vi "RemoveClassesFromTypeDescriptor.vi"(1 "type descriptor":u8[](array[numeric]) format="%x", 3 "replace type desc":u8[](array[numeric])) -> (15 "type descriptor out":u8[](array[numeric]), 18 "type descriptor parsed out":cluster{"TypeDescr":u8[], "Class":bool}[](array[cluster]))   [LabVIEW 2017, in "G#DebugServer.lvclass"]
uses:
  <vilib>/addons/_AddQ/G#DebugServer/G#DebugServer.lvclass
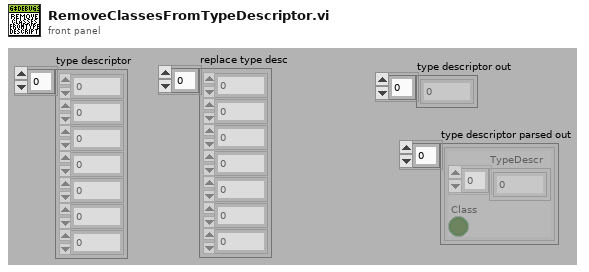
[diagram p1: front panel]
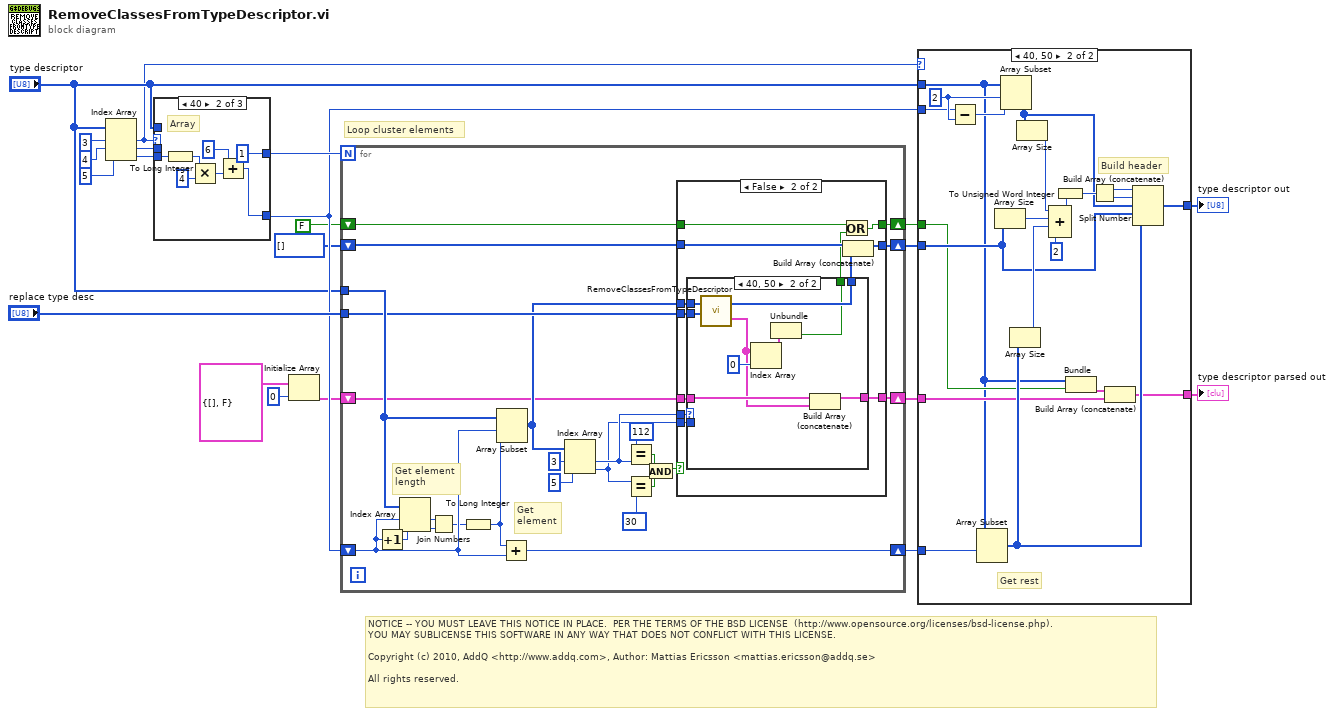
[diagram p0: block diagram]
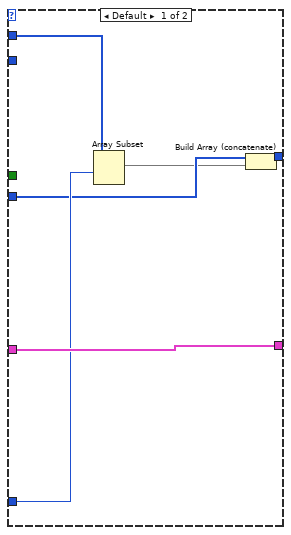
[diagram p2: hidden frame]
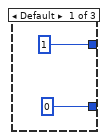
[diagram p3: hidden frame]
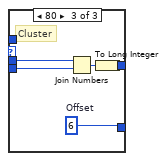
[diagram p4: hidden frame]
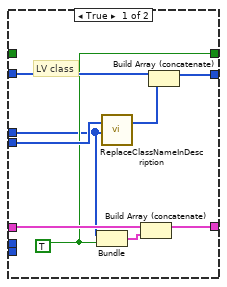
[diagram p5: hidden frame]
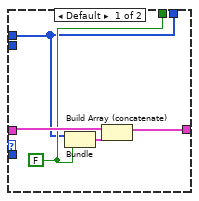
[diagram p6: hidden frame]
diagram:
  # "NOTICE -- YOU MUST LEAVE THIS NOTICE IN PLACE.  PER THE TERMS OF THE BSD LICENSE  (http://www.opensource.org/licenses/bsd-license.php).\nYOU MAY SUBLICENSE THIS SOFTWARE IN ANY WAY THAT DOES NOT CONFLICT WITH THIS LICENSE.\n\nCopyright (c) 2010, AddQ <http://www.addq.com>, Author: Mattias Ericsson <mattias.ericsson@addq.se>\n\nAll rights reserved."
  # "Loop cluster elements"
  n1 = Index Array(array="type descriptor", index #1=3 ("index"), index #2=4 ("index"), index #3=5 ("index")) -> (element #1=w8:u8, element #2=w14:u8, element #3=w9:u8)
  n2 = case shown="40" w8 {
    tunnel: [1 1 w34] -> w18
    tunnel: "type descriptor" -> [_ _ _]
    tunnel: [0 ("Offset") w24 w33] -> w17
    tunnel: w14 -> [_ _ w32]
    tunnel: w9 -> [_ w26 w31]
    frame Default {
    }
    frame 64 {
      # "Array"
      n3 = To Long Integer(number=w26) -> (32bit integer=w30:i32)
      n4 = Multiply(x=w30, y=4) -> (x*y=w28:i32)
      n5 = Add(x=6, y=w28) -> (x+y=w24:i32)
    }
    frame 80 {
      w33 = 6  # Offset
      # "Cluster"
      n6 = Join Numbers(hi=w32, lo=w31) -> ((hi.lo)=w35:u16)
      n7 = To Long Integer(number=w35) -> (32bit integer=w34:i32)
    }
  }
  n8 = Initialize Array(cluster{"TypeDescr":u8[], "Class":bool} {"TypeDescr"=[], "Class"=FALSE}, 0 ("dimension size")) -> (w10:cluster{"TypeDescr":u8[], "Class":bool}[])
  n9 = for {
    N: w18 -> [_]
    tunnel: "type descriptor" -> [w60]
    shift-right: [w59] -> w21
    shift-left: w17 -> [w55]
    shift-right: [w53] -> w12
    shift-left: u8[] [] -> [w54]
    tunnel: "replace type desc" -> [w45]
    shift-right: [w38] -> w7
    shift-left: w10 -> [w39]
    shift-right: [w36] -> w2
    shift-left: FALSE -> [w37]
    # "Get\nelement"
    # "Get element\nlength"
    n10 = Increment(x=w55) -> (x+1=w56:i32)
    n11 = Index Array(array=w60, index #1=w55, index #2=w56) -> (element #1=w57:u8, element #2=w58:u8)
    n12 = Join Numbers(hi=w57, lo=w58) -> ((hi.lo)=w52:u16)
    n13 = To Long Integer(number=w52) -> (32bit integer=w51:i32)
    n14 = Array Subset(array=w60, index=w55, length=w51) -> (w43:u8[])
    n15 = Add(x=w51, y=w55) -> (x+y=w59:i32)
    n16 = Index Array(array=w43, index #1=3 ("index"), index #2=5 ("index")) -> (element #1=w44:u8, element #2=w42:u8)
    n17 = Equal?(x=u8 112 ("element"), y=w44) -> (x = y?=w48:bool)
    n18 = Equal?(x=w42, y=u8 30 ("element")) -> (x = y?=w47:bool)
    n19 = And(x=w48, y=w47) -> (x .and. y?=w46:bool)
    n20 = case shown="False" w46 {
      tunnel: w43 -> [w61 w78]
      tunnel: w54 -> [w69 w81]
      tunnel: [w68 w80] -> w53
      tunnel: w44 -> [_ w79]
      tunnel: w42 -> [_ w77]
      tunnel: w45 -> [w67 w76]
      tunnel: w39 -> [w66 w75]
      tunnel: [w65 w74] -> w38
      tunnel: w37 -> [_ w73]
      tunnel: [w62 w71] -> w36
      frame True {
        w62 = TRUE
        # "LV class"
        n21 = Bundle(w61, w62) -> (w63:cluster{u8[], bool})  [unwired: 1 in]
        n22 = call <vilib>:"ReplaceClassNameInDescription.vi"("replace type descr"=w67, "org class type descr"=w61) -> ("class type decr out"=w64:u8[])  [unwired: 17 in]
        n23 = Build Array (concatenate)(w66, w63) -> (w65:cluster{"TypeDescr":u8[], "Class":bool}[])
        n24 = Build Array (concatenate)(w69, w64) -> (w68:u8[])
      }
      frame False {
        n25 = case shown="40, 50" w79 {
          tunnel: w78 -> [w82 w95]
          tunnel: [w82 w93] -> w70
          tunnel: w77 -> [_ _]
          tunnel: w76 -> [_ w94]
          tunnel: [w86 w91] -> w74
          tunnel: w75 -> [w85 w92]
          tunnel: [w83 w89] -> w72
          frame Default {
            w83 = FALSE
            n26 = Bundle(w82, w83) -> (w84:cluster{u8[], bool})  [unwired: 1 in]
            n27 = Build Array (concatenate)(w85, w84) -> (w86:cluster{"TypeDescr":u8[], "Class":bool}[])
          }
          frame 64, 80 {
            n28 = call <vilib>:"RemoveClassesFromTypeDescriptor.vi"("type descriptor"=w95, "replace type desc"=w94) -> ("type descriptor out"=w93:u8[], "type descriptor parsed out"=w88:cluster{"TypeDescr":u8[], "Class":bool}[])  [unwired: 16 in]
            n29 = Index Array(array=w88, index=0) -> (element=w87:cluster{"TypeDescr":u8[], "Class":bool})
            n30 = Unbundle(w87) -> ("Class"=w89:bool)  [unwired: 1 out]
            n31 = Build Array (concatenate)(w92, w88) -> (w91:cluster{"TypeDescr":u8[], "Class":bool}[])
          }
        }
        n32 = Or(x=w73, y=w72) -> (x .or. y?=w71:bool)
        n33 = Build Array (concatenate)(w81, w70) -> (w80:u8[])
      }
    }
  }
  n34 = case shown="40, 50" w8 {
    tunnel: w21 -> [w99 w122]
    tunnel: w17 -> [_ w110]
    tunnel: "type descriptor" -> [w100 w102]
    tunnel: w12 -> [w98 w108]
    tunnel: [w96 w104] -> w11
    tunnel: w7 -> [w101 w106]
    tunnel: [w101 w107] -> w6
    tunnel: w2 -> [_ w103]
    frame Default {
      n35 = Array Subset(array=w100, index=w99) -> (w97:u8[])  [unwired: 1 in]
      n36 = Build Array (concatenate)(w98, w97) -> (w96:u8[])
    }
    frame 64, 80 {
      w112 = 2 ("index")
      # "Build header"
      # "Get rest"
      n37 = Subtract(x=w110, y=w112) -> (x-y=w111:i32)
      n38 = Array Subset(array=w102, index=w122) -> (w109:u8[])  [unwired: 1 in]
      n39 = Array Size(array=w108) -> (size(s)=w117:i32)
      n40 = Array Subset(array=w102, index=w112, length=w111) -> (w113:u8[])
      n41 = Array Size(array=w109) -> (size(s)=w116:i32)
      n42 = Array Size(array=w113) -> (size(s)=w118:i32)
      n43 = Compound Arithmetic op=ADD(w118, w117, w116, 2 ("value")) -> (w119:i32)
      n44 = To Unsigned Word Integer(number=w119) -> (unsigned 16bit integer=w114:u16)
      n45 = Bundle("type descriptor"=w102, w103) -> (w105:cluster{"type descriptor":u8[], bool})  [unwired: 1 in]
      n46 = Split Number(x=w114) -> (hi(x)=w121:u8, lo(x)=w120:u8)
      n47 = Build Array (concatenate)(w105, w106) -> (w107:cluster{"TypeDescr":u8[], "Class":bool}[])
      n48 = Build Array (concatenate)(w121, w120, w113, w108, w109) -> (w104:u8[])
    }
  }
  "type descriptor out" <- w11
  "type descriptor parsed out" <- w6
